vi "DLP_Two_Colors_ppp.vi"() -> ()   [LabVIEW 2018]
uses:
  mc_api/mc_api.dll
panel:
  out "Second LaserLight On 2":bool
  in  "mode":dbl=1.0
  in  "zero":dbl
  in  "Second Laser Name":i32(ring)=2 items=["Blue", "Green", "Red"]
  in  "First Laser Name":i32(ring) items=["Blue", "Green", "Red"]
  out "DLP on":bool
  in  "Status":dbl
  in  "Second Laser Digital I/O Channel":i32=6
  out "First Laser Light On":bool
  in  "Second LaserTrigger Time(s)":dbl=5.0
  out "Second LaserLight On":bool
  in  "Delay Time (s)":dbl=1.0
  in  "Stop Vi":bool
  in  "First LaserTrigger Time (s)":dbl
  out "error out":errorcluster
  in  "First LaserDigital I/O Channel":i32=7
  in  "Start?":bool
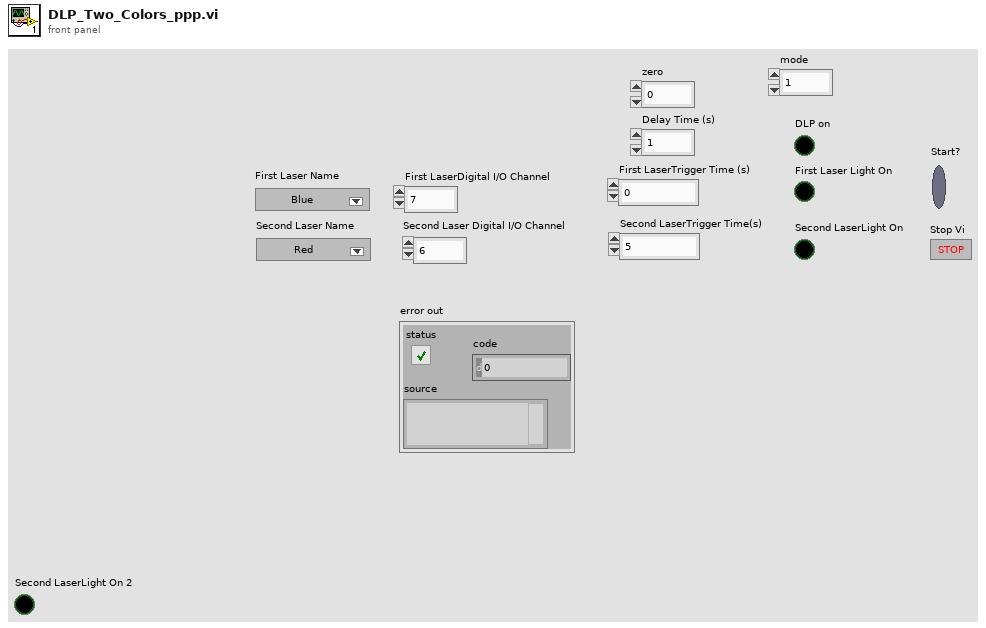
[diagram p1: front panel]
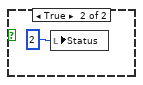
[diagram p3: hidden frame]
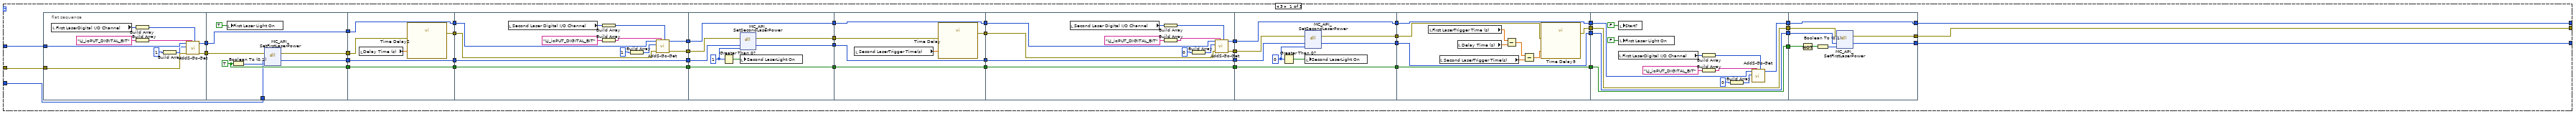
[diagram p4: hidden frame]
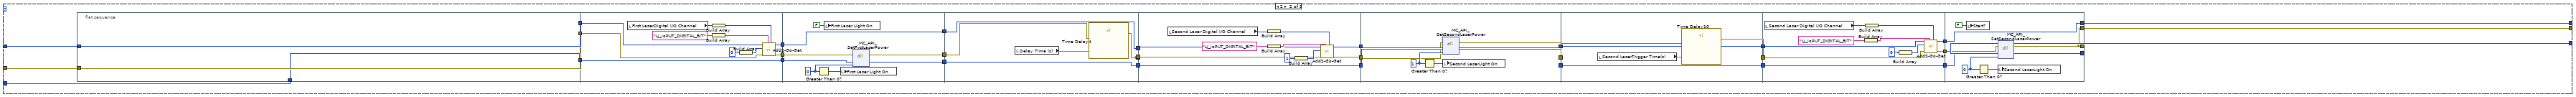
[diagram p5: hidden frame]
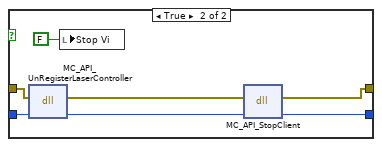
[diagram p6: hidden frame]
diagram:
  n1 = call "configure do to DAC1.vi"() -> ("error out"=w6:errorcluster, "Handle Out"=w1:i32)  [unwired: 10 out]
  n2 = dll-call lib="C:/old/work_pace/mindcontrol_labview/mc_api/mc_api.dll" fn="MC_API_StartClient"(error in=w6) -> (error out=w3:errorcluster, "return type"=w4:i32)  [unwired: 2 in, 1 out]
  n3 = dll-call lib="C:/old/work_pace/mindcontrol_labview/mc_api/mc_api.dll" fn="MC_API_RegisterLaserController"(error in=w3, "sm"=w4) -> (error out=w2:errorcluster, "sm"=w5:i32)  [unwired: 3 in, 1 out]
  n4 = local write "error out"(w2) -> ()
  n5 = while {
    shift-right: [w10] -> _
    shift-left: w2 -> [w7]
    shift-right: [w19] -> _
    shift-left: w5 -> [w8]
    shift-right: [w18] -> _
    shift-left: w1 -> [w9]
    stop <- w11 stop-if-true
    n6 = flat-sequence {
      tunnel: [w24] -> w17
      tunnel: [w27] -> w16
      tunnel: [w20] -> w15
      tunnel: [w26] -> w14
      tunnel: w9 -> [w25]
      tunnel: w8 -> [w23]
      tunnel: w7 -> [w22]
      tunnel: [w369] -> w18
      tunnel: [w368] -> w10
      tunnel: [w365] -> w19
      tunnel: [w370] -> w12
      tunnel: w17 -> [w370]
      tunnel: w16 -> [w366]
      tunnel: w15 -> [w367]
      tunnel: w14 -> [w369]
      tunnel: ["Stop Vi"] -> w13
      frame #0 {
        n7 = local read "Start?"() -> (w21:bool)
        n8 = case shown="真" w21 {
          tunnel: [w30 w45] -> w27
          tunnel: [w29 w50] -> w26
          tunnel: w25 -> [w29 w47]
          tunnel: w23 -> [w30 w48]
          tunnel: w22 -> [w28 w49]
          tunnel: [w28 w43] -> w20
          frame False {
          }
          frame True {
            n9 = flat-sequence {
              tunnel: w49 -> [w358]
              tunnel: [w361] -> w35
              tunnel: w48 -> [w360]
              tunnel: [w359] -> w33
              tunnel: [w357] -> w37
              tunnel: w47 -> [w357]
              frame #0 {
                w363 = 1
                n10 = dll-call lib="C:/old/work_pace/mindcontrol_labview/mc_api/mc_api.dll" fn="MC_API_SetDLPOnOff"(error in=w358, "sm"=w360, "g"=w363) -> (error out=w361:errorcluster, "sm"=w359:i32)  [unwired: 4 in, 1 out]
                n11 = Greater Than 0?(x=w363) -> (x > 0?=w362:bool)
                n12 = local write "DLP on"(w362) -> ()
              }
            }
            n13 = stacked-sequence {
              tunnel: [w62] -> w38
              tunnel: w37 -> [w62]
              tunnel: w35 -> [w61]
              tunnel: [w60] -> w34
              tunnel: w33 -> [w59]
              tunnel: [w58] -> w32
              frame #0 {
                n14 = local read "First Laser Name"() -> (w57:i32)
                n15 = dll-call lib="C:/old/work_pace/mindcontrol_labview/mc_api/mc_api.*" fn="MC_API_SetFirstLaserName"(error in=w61, "sm"=w59, "name"=w57) -> (error out=w60:errorcluster, "sm"=w58:i32)  [unwired: 4 in, 1 out]
              }
            }
            n16 = stacked-sequence {
              tunnel: [w53] -> w39
              tunnel: w38 -> [w53]
              tunnel: [w51] -> w36
              tunnel: w34 -> [w52]
              tunnel: w32 -> [w55]
              tunnel: [w54] -> w31
              frame #0 {
                n17 = local read "Second Laser Name"() -> (w56:i32)
                n18 = dll-call lib="C:/old/work_pace/mindcontrol_labview/mc_api/mc_api.*" fn="MC_API_SetSecondLaserName"(error in=w52, "sm"=w55, "name"=w56) -> (error out=w51:errorcluster, "sm"=w54:i32)  [unwired: 4 in, 1 out]
              }
            }
            n19 = flat-sequence {
              tunnel: w36 -> [w66]
              tunnel: w31 -> [w67]
              tunnel: w39 -> [w68]
              tunnel: [w68] -> w42
              tunnel: [w67] -> w41
              tunnel: [w66] -> w40
              tunnel: [w77] -> w46
              tunnel: [w76] -> w50
              tunnel: w42 -> [w75]
              tunnel: w41 -> [w74]
              tunnel: w40 -> [w73]
              tunnel: [w71] -> w44
              frame #0 {
                n20 = local read "mode"() -> (w63:dbl)
                n21 = Greater?(x=w63, y=1) -> (0:w65:bool)
                n22 = case shown="假" w65 {
                  frame False {
                    n23 = local write "Status"(1) -> ()
                  }
                  frame True {
                    n24 = local write "Status"(2) -> ()
                  }
                }
              }
              frame #1 {
                n25 = local read "Status"() -> (w72:dbl)
                n26 = case shown="1, 默认" w72 {
                  tunnel: [w112 w250 w325] -> w77
                  tunnel: [w121 w249 w324] -> w76
                  tunnel: w75 -> [w120 w253 w333]
                  tunnel: w74 -> [w119 w252 w332]
                  tunnel: w73 -> [w118 w251 w331]
                  tunnel: [w78 w236 w323] -> w71
                  frame 3 {
                    n27 = flat-sequence {
                      tunnel: w120 -> [w129]
                      tunnel: [w126] -> w110
                      tunnel: w118 -> [w125]
                      tunnel: [w124] -> w109
                      tunnel: [w135] -> w117
                      tunnel: [w138] -> w116
                      tunnel: w119 -> [w137]
                      tunnel: [w136] -> w115
                      tunnel: [w134] -> w111
                      tunnel: w110 -> [w134]
                      tunnel: w109 -> [w133]
                      tunnel: w117 -> [w145]
                      tunnel: w116 -> [w141]
                      tunnel: w115 -> [w143]
                      tunnel: w111 -> [w142]
                      tunnel: [w144] -> w102
                      tunnel: [w143] -> w101
                      tunnel: [w142] -> w99
                      tunnel: [w141] -> w97
                      tunnel: w102 -> [w149]
                      tunnel: w101 -> [w157]
                      tunnel: [w157] -> w100
                      tunnel: w99 -> [w147]
                      tunnel: [w146] -> w98
                      tunnel: w97 -> [w156]
                      tunnel: [w156] -> w96
                      tunnel: [w148] -> w95
                      tunnel: [w160] -> w114
                      tunnel: [w158] -> w113
                      tunnel: w100 -> [w159]
                      tunnel: [w164] -> w105
                      tunnel: w98 -> [w164]
                      tunnel: [w163] -> w103
                      tunnel: w96 -> [w163]
                      tunnel: w95 -> [w161]
                      tunnel: w114 -> [w171]
                      tunnel: [w170] -> w94
                      tunnel: [w169] -> w92
                      tunnel: w113 -> [w169]
                      tunnel: [w168] -> w90
                      tunnel: w105 -> [w168]
                      tunnel: [w167] -> w88
                      tunnel: w103 -> [w167]
                      tunnel: w94 -> [w173]
                      tunnel: [w172] -> w93
                      tunnel: w92 -> [w183]
                      tunnel: [w183] -> w91
                      tunnel: w90 -> [w175]
                      tunnel: [w174] -> w89
                      tunnel: w88 -> [w182]
                      tunnel: [w182] -> w87
                      tunnel: w93 -> [w188]
                      tunnel: w91 -> [w185]
                      tunnel: [w187] -> w86
                      tunnel: [w186] -> w84
                      tunnel: [w190] -> w82
                      tunnel: w89 -> [w190]
                      tunnel: [w189] -> w80
                      tunnel: w87 -> [w189]
                      tunnel: w86 -> [w193]
                      tunnel: [w192] -> w85
                      tunnel: w84 -> [w201]
                      tunnel: [w201] -> w83
                      tunnel: w82 -> [w200]
                      tunnel: [w200] -> w81
                      tunnel: w80 -> [w199]
                      tunnel: [w199] -> w79
                      tunnel: w85 -> [w214]
                      tunnel: w83 -> [w213]
                      tunnel: [w214] -> w108
                      tunnel: [w212] -> w107
                      tunnel: [w213] -> w106
                      tunnel: w81 -> [w211]
                      tunnel: [w210] -> w104
                      tunnel: w79 -> [w210]
                      tunnel: [w215] -> w112
                      tunnel: [w222] -> w121
                      tunnel: [w217] -> w78
                      tunnel: w108 -> [w218]
                      tunnel: w107 -> [w222]
                      tunnel: w106 -> [w216]
                      tunnel: w104 -> [w219]
                      frame #0 {
                        n28 = local read "First LaserDigital I/O Channel"() -> (w127:i32)
                        n29 = Build Array(w127) -> (w128:i32[])
                        n30 = Build Array("LJ_ioPUT_DIGITAL_BIT" ("IOType")) -> (w130:string[])
                        n31 = Build Array(1) -> (w122:i32[])
                        n32 = call "AddS-Go-Get.vi"("Channels"=w128, "IOTypes"=w130, "error in"=w125, "Values Write"=w122, "Handle In"=w129) -> ("error out"=w124:errorcluster, "Handle Out"=w126:i32)  [unwired: 4 in, 1 out]
                      }
                      frame #1 {
                        w138 = TRUE
                        n33 = local write "First Laser Light On"(TRUE) -> ()
                        n34 = Boolean To (0,1)(Boolean=w138) -> (0, 1=w139:i16)
                        n35 = dll-call lib="C:/old/work_pace/mindcontrol_labview/mc_api/mc_api.dll" fn="MC_API_SetFirstLaserPower"(error in=w133, "sm"=w137, "g"=w139) -> (error out=w135:errorcluster, "sm"=w136:i32)  [unwired: 4 in, 1 out]
                      }
                      frame #2 {
                        n36 = local read "Delay Time (s)"() -> (w140:dbl)
                        n37 = call "Time Delay2"("error in (no error)"=w145, "Delay Time (s)"=w140) -> ("error out"=w144:errorcluster)  [unwired: 9 in]
                      }
                      frame #3 {
                        n38 = local read "Second Laser Digital I/O Channel"() -> (w153:i32)
                        n39 = Build Array(w153) -> (w152:i32[])
                        n40 = Build Array("LJ_ioPUT_DIGITAL_BIT" ("IOType")) -> (w151:string[])
                        n41 = Build Array(1) -> (w155:i32[])
                        n42 = call "AddS-Go-Get.vi"("Channels"=w152, "IOTypes"=w151, "error in"=w149, "Values Write"=w155, "Handle In"=w147) -> ("error out"=w148:errorcluster, "Handle Out"=w146:i32)  [unwired: 4 in, 1 out]
                      }
                      frame #4 {
                        w162 = 1
                        n43 = Greater Than 0?(x=w162) -> (x > 0?=w165:bool)
                        n44 = dll-call lib="C:/old/work_pace/mindcontrol_labview/mc_api/mc_api.dll" fn="MC_API_SetSecondLaserPower"(error in=w161, "sm"=w159, "g"=w162) -> (error out=w160:errorcluster, "sm"=w158:i32)  [unwired: 4 in, 1 out]
                        n45 = local write "Second LaserLight On"(w165) -> ()
                      }
                      frame #5 {
                        n46 = local read "Second LaserTrigger Time(s)"() -> (w166:dbl)
                        n47 = call "Time Delay"("error in (no error)"=w171, "Delay Time (s)"=w166) -> ("error out"=w170:errorcluster)  [unwired: 9 in]
                      }
                      frame #6 {
                        n48 = local read "Second Laser Digital I/O Channel"() -> (w178:i32)
                        n49 = Build Array(w178) -> (w179:i32[])
                        n50 = Build Array("LJ_ioPUT_DIGITAL_BIT" ("IOType")) -> (w180:string[])
                        n51 = Build Array(0) -> (w176:i32[])
                        n52 = call "AddS-Go-Get.vi"("Channels"=w179, "IOTypes"=w180, "error in"=w173, "Values Write"=w176, "Handle In"=w175) -> ("error out"=w172:errorcluster, "Handle Out"=w174:i32)  [unwired: 4 in, 1 out]
                      }
                      frame #7 {
                        w184 = 0
                        n53 = Greater Than 0?(x=w184) -> (x > 0?=w191:bool)
                        n54 = dll-call lib="C:/old/work_pace/mindcontrol_labview/mc_api/mc_api.dll" fn="MC_API_SetSecondLaserPower"(error in=w188, "sm"=w185, "g"=w184) -> (error out=w187:errorcluster, "sm"=w186:i32)  [unwired: 4 in, 1 out]
                        n55 = local write "Second LaserLight On"(w191) -> ()
                      }
                      frame #8 {
                        n56 = local read "First LaserTrigger Time (s)"() -> (w198:dbl)
                        n57 = local read "Second LaserTrigger Time(s)"() -> (w195:dbl)
                        n58 = local read "Delay Time (s)"() -> (w197:dbl)
                        n59 = Subtract(x=w198, y=w197) -> (x-y=w196:dbl)
                        n60 = Subtract(x=w196, y=w195) -> (x-y=w194:dbl)
                        n61 = call "Time Delay9"("error in (no error)"=w193, "Delay Time (s)"=w194) -> ("error out"=w192:errorcluster)  [unwired: 9 in]
                      }
                      frame #9 {
                        n62 = local read "First LaserDigital I/O Channel"() -> (w207:i32)
                        n63 = local write "Start?"(FALSE) -> ()
                        n64 = local write "First Laser Light On"(FALSE) -> ()
                        n65 = Build Array(w207) -> (w205:i32[])
                        n66 = Build Array("LJ_ioPUT_DIGITAL_BIT" ("IOType")) -> (w204:string[])
                        n67 = Build Array(0) -> (w208:i32[])
                        n68 = call "AddS-Go-Get.vi"("Channels"=w205, "IOTypes"=w204, "Values Write"=w208, "Handle In"=w211) -> ("Handle Out"=w212:i32)  [unwired: 5 in, 2 out]
                      }
                      frame #10 {
                        n69 = Not(x=w219) -> (.not. x?=w220:bool)
                        n70 = Boolean To (0,1)(Boolean=w220) -> (0, 1=w221:i16)
                        n71 = dll-call lib="C:/old/work_pace/mindcontrol_labview/mc_api/mc_api.dll" fn="MC_API_SetFirstLaserPower"(error in=w218, "sm"=w216, "g"=w221) -> (error out=w217:errorcluster, "sm"=w215:i32)  [unwired: 4 in, 1 out]
                      }
                    }
                  }
                  frame 2 {
                    n72 = flat-sequence {
                      tunnel: [w255] -> w245
                      tunnel: [w254] -> w243
                      tunnel: [w256] -> w240
                      tunnel: w253 -> [w256]
                      tunnel: w251 -> [w255]
                      tunnel: w252 -> [w254]
                      tunnel: w245 -> [w258]
                      tunnel: [w257] -> w244
                      tunnel: w243 -> [w267]
                      tunnel: [w267] -> w242
                      tunnel: [w259] -> w241
                      tunnel: w240 -> [w260]
                      tunnel: w244 -> [w272]
                      tunnel: [w271] -> w248
                      tunnel: w242 -> [w274]
                      tunnel: [w273] -> w247
                      tunnel: w241 -> [w275]
                      tunnel: [w275] -> w246
                      tunnel: w248 -> [w280]
                      tunnel: [w277] -> w235
                      tunnel: [w279] -> w234
                      tunnel: w247 -> [w279]
                      tunnel: [w278] -> w233
                      tunnel: w246 -> [w278]
                      tunnel: [w277] -> w232
                      tunnel: w235 -> [_]
                      tunnel: [w281] -> w231
                      tunnel: w234 -> [w291]
                      tunnel: [w291] -> w230
                      tunnel: w233 -> [w284]
                      tunnel: [w283] -> w229
                      tunnel: w232 -> [w282]
                      tunnel: w231 -> [w293]
                      tunnel: [w292] -> w228
                      tunnel: w230 -> [w295]
                      tunnel: [w294] -> w226
                      tunnel: w229 -> [w296]
                      tunnel: [w296] -> w224
                      tunnel: w228 -> [w300]
                      tunnel: [w299] -> w227
                      tunnel: w226 -> [w303]
                      tunnel: [w303] -> w225
                      tunnel: w224 -> [w302]
                      tunnel: [w302] -> w223
                      tunnel: w227 -> [w305]
                      tunnel: [w304] -> w239
                      tunnel: w225 -> [w314]
                      tunnel: [w314] -> w238
                      tunnel: w223 -> [w307]
                      tunnel: [w306] -> w237
                      tunnel: w239 -> [w319]
                      tunnel: w238 -> [w318]
                      tunnel: [w321] -> w249
                      tunnel: [w316] -> w250
                      tunnel: [w315] -> _
                      tunnel: w237 -> [w321]
                      tunnel: [w315] -> w236
                      frame #0 {
                      }
                      frame #1 {
                        n73 = local read "First LaserDigital I/O Channel"() -> (w264:i32)
                        n74 = Build Array(w264) -> (w262:i32[])
                        n75 = Build Array("LJ_ioPUT_DIGITAL_BIT" ("IOType")) -> (w261:string[])
                        n76 = Build Array(0) -> (w265:i32[])
                        n77 = call "AddS-Go-Get.vi"("Channels"=w262, "IOTypes"=w261, "error in"=w258, "Values Write"=w265, "Handle In"=w260) -> ("error out"=w257:errorcluster, "Handle Out"=w259:i32)  [unwired: 4 in, 1 out]
                      }
                      frame #2 {
                        w268 = 0
                        n78 = Greater Than 0?(x=w268) -> (x > 0?=w269:bool)
                        n79 = local write "First Laser Light On"(FALSE) -> ()
                        n80 = local write "First Laser Light On"(w269) -> ()
                        n81 = dll-call lib="C:/old/work_pace/mindcontrol_labview/mc_api/mc_api.dll" fn="MC_API_SetFirstLaserPower"(error in=w272, "sm"=w274, "g"=w268) -> (error out=w271:errorcluster, "sm"=w273:i32)  [unwired: 4 in, 1 out]
                      }
                      frame #3 {
                        n82 = local read "Delay Time (s)"() -> (w276:dbl)
                        n83 = call "Time Delay4"("error in (no error)"=w280, "Delay Time (s)"=w276) -> ("error out"=w277:errorcluster)  [unwired: 9 in]
                      }
                      frame #4 {
                        n84 = local read "Second Laser Digital I/O Channel"() -> (w289:i32)
                        n85 = Build Array(w289) -> (w287:i32[])
                        n86 = Build Array("LJ_ioPUT_DIGITAL_BIT" ("IOType")) -> (w290:string[])
                        n87 = Build Array(1) -> (w288:i32[])
                        n88 = call "AddS-Go-Get.vi"("Channels"=w287, "IOTypes"=w290, "error in"=w282, "Values Write"=w288, "Handle In"=w284) -> ("error out"=w281:errorcluster, "Handle Out"=w283:i32)  [unwired: 4 in, 1 out]
                      }
                      frame #5 {
                        w297 = 1
                        n89 = Greater Than 0?(x=w297) -> (x > 0?=w298:bool)
                        n90 = dll-call lib="C:/old/work_pace/mindcontrol_labview/mc_api/mc_api.dll" fn="MC_API_SetSecondLaserPower"(error in=w293, "sm"=w295, "g"=w297) -> (error out=w292:errorcluster, "sm"=w294:i32)  [unwired: 4 in, 1 out]
                        n91 = local write "Second LaserLight On"(w298) -> ()
                      }
                      frame #6 {
                        n92 = local read "Second LaserTrigger Time(s)"() -> (w301:dbl)
                        n93 = call "Time Delay10"("error in (no error)"=w300, "Delay Time (s)"=w301) -> ("error out"=w299:errorcluster)  [unwired: 9 in]
                      }
                      frame #7 {
                        n94 = local read "Second Laser Digital I/O Channel"() -> (w310:i32)
                        n95 = Build Array("LJ_ioPUT_DIGITAL_BIT" ("IOType")) -> (w312:string[])
                        n96 = Build Array(w310) -> (w311:i32[])
                        n97 = Build Array(0) -> (w308:i32[])
                        n98 = call "AddS-Go-Get.vi"("Channels"=w311, "IOTypes"=w312, "error in"=w305, "Values Write"=w308, "Handle In"=w307) -> ("error out"=w304:errorcluster, "Handle Out"=w306:i32)  [unwired: 4 in, 1 out]
                      }
                      frame #8 {
                        w317 = 0
                        n99 = local write "Start?"(FALSE) -> ()
                        n100 = Greater Than 0?(x=w317) -> (x > 0?=w322:bool)
                        n101 = dll-call lib="C:/old/work_pace/mindcontrol_labview/mc_api/mc_api.dll" fn="MC_API_SetSecondLaserPower"(error in=w319, "sm"=w318, "g"=w317) -> (error out=w315:errorcluster, "sm"=w316:i32)  [unwired: 4 in, 1 out]
                        n102 = local write "Second LaserLight On"(w322) -> ()
                      }
                    }
                  }
                  frame 1, Default {
                    n103 = flat-sequence {
                      tunnel: w333 -> [w341]
                      tunnel: [w338] -> w330
                      tunnel: w331 -> [w337]
                      tunnel: [w336] -> w329
                      tunnel: [w349] -> w328
                      tunnel: w332 -> [w351]
                      tunnel: [w350] -> w327
                      tunnel: [w348] -> w326
                      tunnel: w330 -> [w348]
                      tunnel: w329 -> [w347]
                      tunnel: [w354] -> w324
                      tunnel: [w352] -> w325
                      tunnel: [w353] -> w323
                      tunnel: w326 -> [w354]
                      tunnel: w327 -> [w352]
                      tunnel: w328 -> [w353]
                      frame #0 {
                        n104 = local read "First LaserDigital I/O Channel"() -> (w339:i32)
                        n105 = Build Array(w339) -> (w340:i32[])
                        n106 = Build Array("LJ_ioPUT_DIGITAL_BIT" ("IOType")) -> (w342:string[])
                        n107 = Build Array(1) -> (w334:i32[])
                        n108 = call "AddS-Go-Get.vi"("Channels"=w340, "IOTypes"=w342, "error in"=w337, "Values Write"=w334, "Handle In"=w341) -> ("error out"=w336:errorcluster, "Handle Out"=w338:i32)  [unwired: 4 in, 1 out]
                      }
                      frame #1 {
                        w344 = 1
                        n109 = Greater Than 0?(x=w344) -> (x > 0?=w345:bool)
                        n110 = local write "First Laser Light On"(w345) -> ()
                        n111 = dll-call lib="C:/old/work_pace/mindcontrol_labview/mc_api/mc_api.dll" fn="MC_API_SetFirstLaserPower"(error in=w347, "sm"=w351, "g"=w344) -> (error out=w349:errorcluster, "sm"=w350:i32)  [unwired: 4 in, 1 out]
                        n112 = local write "Start?"(FALSE) -> ()
                      }
                      frame #2 {
                      }
                    }
                  }
                }
              }
            }
            n113 = flat-sequence {
              tunnel: w44 -> [w356]
              tunnel: w46 -> [w355]
              tunnel: [w355] -> w45
              tunnel: [w356] -> w43
              frame #0 {
              }
            }
          }
        }
        n114 = local write "error out"(w20) -> ()
        n115 = Unbundle By Name(w20) -> ("status"=w24:bool)
      }
      frame #1 {
        n116 = case shown="假" "Stop Vi" {
          tunnel: [w372 w377] -> w368
          tunnel: w367 -> [w372 w376]
          tunnel: w366 -> [w371 w375]
          tunnel: [w371 w374] -> w365
          frame False {
          }
          frame True {
            n117 = dll-call lib="C:/old/work_pace/mindcontrol_labview/mc_api/mc_api.dll" fn="MC_API_UnRegisterLaserController"(error in=w376, "sm"=w375) -> (error out=w378:errorcluster, "sm"=w379:i32)  [unwired: 3 in, 1 out]
            n118 = local write "Stop Vi"(FALSE) -> ()
            n119 = dll-call lib="C:/old/work_pace/mindcontrol_labview/mc_api/mc_api.dll" fn="MC_API_StopClient"(error in=w378, "sm"=w379) -> (error out=w377:errorcluster, "sm"=w374:i32)  [unwired: 3 in, 1 out]
          }
        }
      }
    }
    n120 = Or(x=w12, y=w13) -> (x .or. y?=w11:bool)
    n121 = local write "error out"(w10) -> ()
  }
